vi "EditValue.vi"(8 "error in (no error)":errorcluster, 10 "Bounds":T1, 11 "U32 D Element.lvclass":refnum<class "String D Element.lvclass">) -> (0 "error out":errorcluster, 1 "Tabbed out?":bool, 2 "Value changed?":bool, 3 "U32 D Element.lvclass":refnum<class "String D Element.lvclass">)   [LabVIEW 2018, in "D Datagrid Library.lvlib" / "String D Element.lvclass"]
uses:
  String D Element.lvclass
  <vilib>/Utility/miscctls.llb/LVRectTypeDef.ctl
panel:
  in  "Value":string
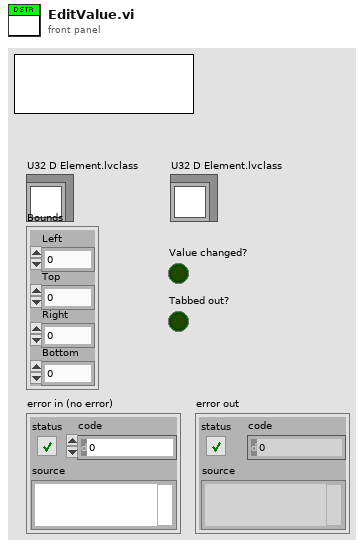
[diagram p1: front panel]
types:
  T1 = typedef "LVRectTypeDef.ctl" = cluster{"Left":i16, "Top":i16, "Right":i16, "Bottom":i16}
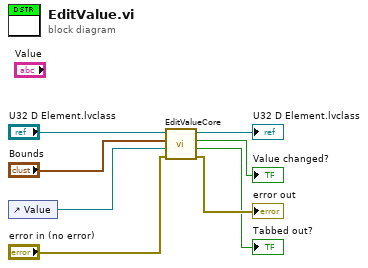
[diagram p0: block diagram]
diagram:
  n1 = control-ref of="Value"() -> (w3:refnum<vi>)
  n2 = call-dynamic "EditValueCore.vi"("error in (no error)"="error in (no error)", "Value field reference"=w3, "Bounds"="Bounds", "DatagridElement in"="U32 D Element.lvclass") -> ("error out"=→"error out":errorcluster, "Tabbed out?"=→"Tabbed out?":bool, "Value changed?"=→"Value changed?":bool, "DatagridElement out"=→"U32 D Element.lvclass":refnum<class "String D Element.lvclass">)  [unwired: 4 in]
